vi "PCI1220U速度设置.vi"(10 "Change Velocity":dbl=10000.0, 11 "AxisHandle IN":u32) -> (3 "AxisHandle OUT":u32)   [LabVIEW 2013]
panel:
  out "ReturnValue":u32
  out "输出变量":dbl
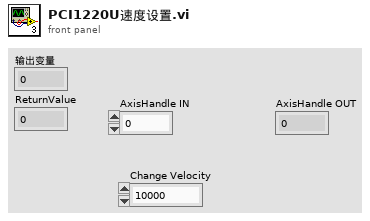
[diagram p1: front panel]
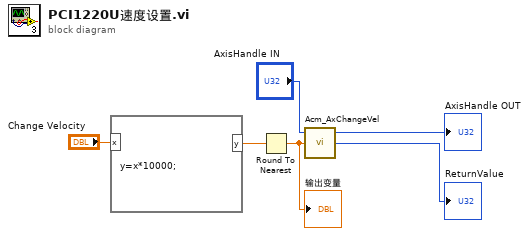
[diagram p0: block diagram]
diagram:
  n1 = formula code="y=x*10000;"("x"="Change Velocity") -> ("y"=w2:dbl)
  n2 = Round To Nearest(number=w2) -> (nearest integer value=w1:dbl)
  "输出变量" <- w1
  n3 = call <userlib>:"Acm_AxChangeVel.vi"("NewVelocity"=w1, "AxisHandle"="AxisHandle IN") -> ("ReturnValue"=→"ReturnValue":u32, "AxisHandle 2"=→"AxisHandle OUT":u32)  [unwired: 1 in, 1 out]
